vi "MultiChannnel_Log.vi"() -> ()   [LabVIEW 2024]
uses:
  <vilib>/DAQmx/read.llb/DAQmx Read (Analog 1D Wfm NChan NSamp).vi
  <vilib>/DAQmx/create/channels.llb/DAQmx Create Channel (AI-Voltage-Basic).vi
  <vilib>/DAQmx/configure/timing.llb/DAQmx Timing (Sample Clock).vi
  <vilib>/DAQmx/miscellaneous.llb/DAQmx Fill In Error Info.vi
  <vilib>/Waveform/WDTOps.llb/WDT Index Channel DBL.vi
panel:
  out "appended array":dbl[][](array[numeric])
  out "Y 3":dbl[](array[numeric])
  out "Y 2":dbl[](array[numeric])
  out "Y":dbl[](array[numeric])
  in  "stop":bool
  out "Waveform Graph":waveform(dbl)[](graph)
  in  "samples per channel":i32=1000
  in  "sample mode":i32(ring)=10178 items=["Finite Samples"=10178, "Continuous Samples"=10123, "Hardware Timed Single Point"=12522]
  in  "rate":dbl=20000.0 format="%0.2f"
  in  "physical channels":tag
  # "Phy Channel -> Set to 0-2\nRate 1000Hz\nSampleMode  -> Contenious Sampling\nSample per Channel -> 100"
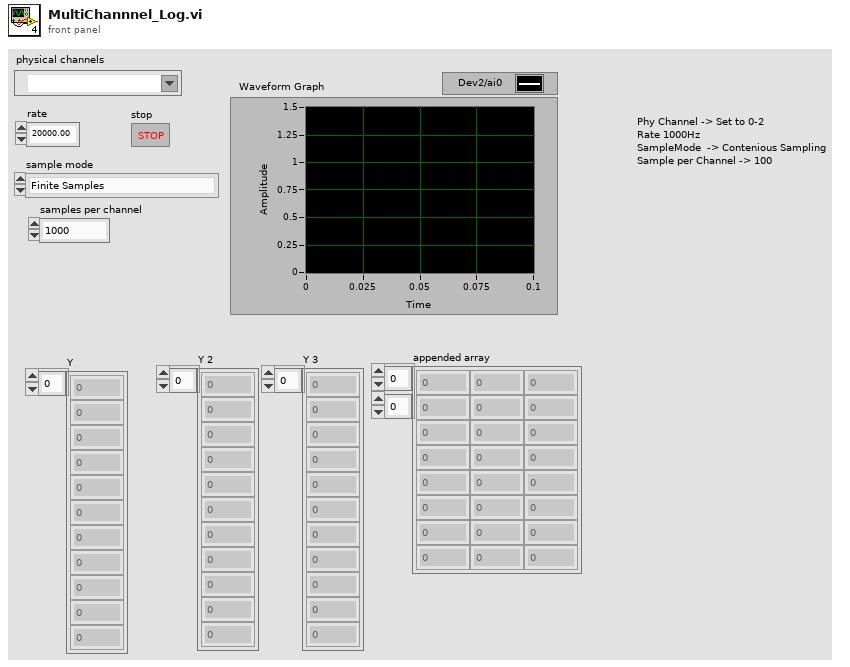
[diagram p1: front panel]
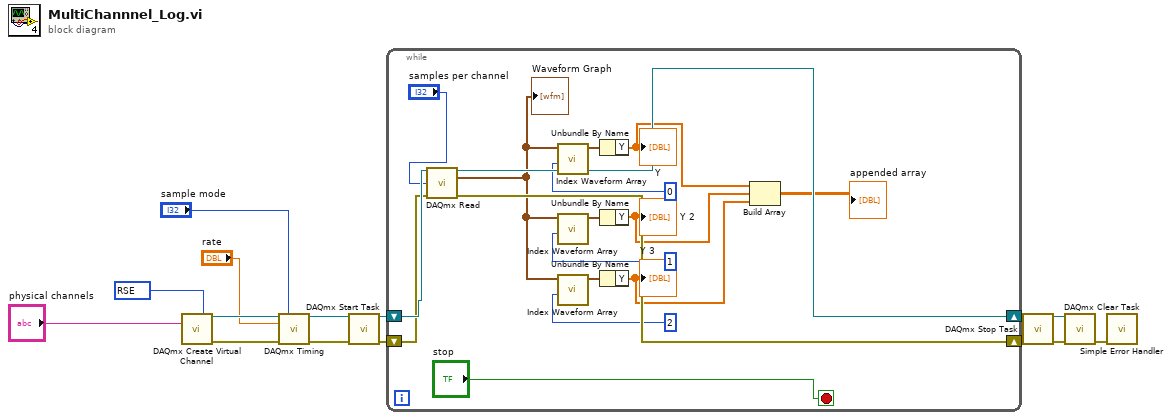
[diagram p0: block diagram]
diagram:
  w1 = 10083 items=["Default"=-1, "RSE"=10083, "NRSE"=10078, "Differential"=10106, "Pseudodifferential"=12529] ("input terminal configuration")
  n1 = call-poly <vilib>:"DAQmx Create Virtual Channel.vi"("input terminal configuration"=w1, "physical channels"="physical channels") -> ("task out"=w7:refnum<k21>, "error out"=w6:errorcluster)  [unwired: 12 in]
  n2 = call-poly <vilib>:"DAQmx Timing.vi"("task/channels in"=w7, "sample mode"="sample mode", "rate"="rate", "error in"=w6) -> ("task out"=w5:refnum<k21>, "error out"=w4:errorcluster)  [unwired: 10 in]
  n3 = call <vilib>:"DAQmx Start Task.vi"("task/channels in"=w5, "error in"=w4) -> ("task out"=w14:refnum<k21>, "error out"=w13:errorcluster)  [unwired: 12 in]
  n4 = while {
    shift-right: [w29] -> w11
    shift-left: w14 -> [w32]
    shift-right: [w30] -> w12
    shift-left: w13 -> [w31]
    stop <- "stop" stop-if-true
    n5 = call-poly <vilib>:"DAQmx Read.vi"("task/channels in"=w32, "number of samples per channel"="samples per channel", "error in"=w31) -> ("task out"=w29:refnum<k21>, "data"=w20:waveform(dbl)[], "error out"=w30:errorcluster)  [unwired: 10 in]
    "Waveform Graph" <- w20
    n6 = call-poly <vilib>:"Index Waveform Array.vi"("index"=0, "waveform array"=w20) -> ("waveform"=w25:waveform(dbl))  [unwired: 8 in, 1 out]
    n7 = call-poly <vilib>:"Index Waveform Array.vi"("index"=1, "waveform array"=w20) -> ("waveform"=w23:waveform(dbl))  [unwired: 8 in, 1 out]
    n8 = call-poly <vilib>:"Index Waveform Array.vi"("index"=2, "waveform array"=w20) -> ("waveform"=w21:waveform(dbl))  [unwired: 8 in, 1 out]
    n9 = Unbundle By Name(w25) -> ("Y"=w19:dbl[])
    "Y" <- w19
    n10 = Unbundle By Name(w23) -> ("Y"=w18:dbl[])
    "Y 2" <- w18
    n11 = Unbundle By Name(w21) -> ("Y"=w17:dbl[])
    "Y 3" <- w17
    n12 = Build Array(w19, w18, w17) -> (→"appended array":dbl[][])
  }
  n13 = call <vilib>:"DAQmx Stop Task.vi"("task/channels in"=w11, "error in"=w12) -> ("task out"=w9:refnum<k21>, "error out"=w10:errorcluster)  [unwired: 12 in]
  n14 = call <vilib>:"DAQmx Clear Task.vi"("task in"=w9, "error in"=w10) -> ("error out"=w8:errorcluster)  [unwired: 13 in]
  n15 = call <vilib>:"Simple Error Handler.vi"("error in (no error)"=w8) -> ()  [unwired: 4 in, 5 out]
